vi "Ref Trig Buffer (Multi-Channel).vi"(0 "data in":u32[](array[numeric])=[0, 0], 1 "reset":bool, 5 "reference trigger":bool, 7 "pretrigger samples":u32, 9 "input valid":bool, 11 "abort":bool) -> (4 "data out":u32[](array[numeric]), 10 "output valid":bool, 13 "ready for reference":bool)   [LabVIEW 2023]
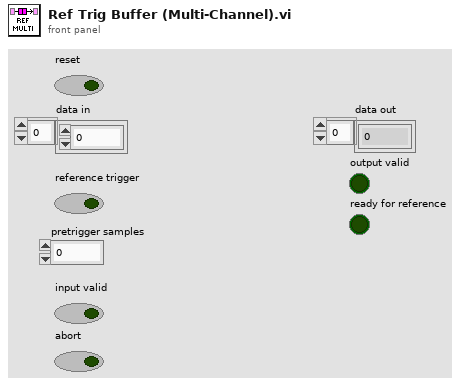
[diagram p1: front panel]
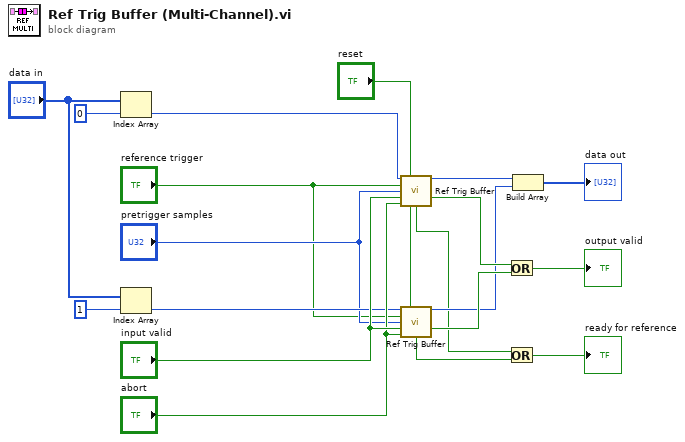
[diagram p0: block diagram]
diagram:
  n1 = Index Array(array="data in", index=0) -> (element=w16:u32)
  n2 = Index Array(array="data in", index=1) -> (element=w4:u32)
  n3 = call <instrlib>:"Ref Trig Buffer.vi"("data in"=w16, "reset"="reset", "reference trigger"="reference trigger", "pretrigger samples"="pretrigger samples", "input valid"="input valid", "abort"="abort") -> ("data out"=w11:u32, "output valid"=w13:bool, "ready for reference"=w7:bool)  [unwired: 7 in]
  n4 = call <instrlib>:"Ref Trig Buffer.vi"("data in"=w4, "reset"="reset", "reference trigger"="reference trigger", "pretrigger samples"="pretrigger samples", "input valid"="input valid", "abort"="abort") -> ("data out"=w10:u32, "output valid"=w12:bool, "ready for reference"=w8:bool)  [unwired: 7 in]
  n5 = Or(x=w13, y=w12) -> (x .or. y?=→"output valid":bool)
  n6 = Or(x=w7, y=w8) -> (x .or. y?=→"ready for reference":bool)
  n7 = Build Array(w11, w10) -> (→"data out":u32[])
